vi "parse.vi"(8 "error in (no error)":errorcluster, 10 "ModbusBuffer in":refnum<class "ModbusBuffer.lvclass">, 11 "ILCCommunications in":refnum<class "ILCCommunications.lvclass">) -> (0 "error out":errorcluster, 2 "ModbusBuffer out":refnum<class "ModbusBuffer.lvclass">, 3 "ILCCommunications out":refnum<class "ILCCommunications.lvclass">)   [LabVIEW 2016, in "ILCCommunications.lvclass"]
uses:
  ILCCommunications.lvclass
  Common_RT_Modbus/ModbusBuffer/ModbusBuffer.lvclass
  Common_RT_Modbus/ModbusBuffer/ModbusBuffer.lvclass/ModbusBuffer.ctl
  ILCCommunications.lvclass/ILCCommunications.ctl
  Common_RT_ILC/ILC/ILC.lvclass/ILC.ctl
  Common_RT_HPILC/HPILC/HPILC.lvclass/HPILC.ctl
  Common_RT_FAILC/FAILC/FAILC.lvclass/FAILC.ctl
  Common_RT_Modbus/ModbusBuffer/readInstructionByte.vi
  getILCMap.vi
  Common_RT_ILC/ILC/parseILC.vi
  Common_RT_HPILC/HPILC/parseStepMotorResponse.vi
  Common_RT_HPILC/HPILC/parseStepMotorError.vi
  Common_RT_HPILC/HPILC/parseForceAndStatusResponse.vi
  Common_RT_HPILC/HPILC/parseForceAndStatusError.vi
  Common_RT_FAILC/FAILC/parseBoosterValveGainResponse.vi
  Common_RT_FAILC/FAILC/parseBoosterValveGainError.vi
  Common_RT_FAILC/FAILC/parseReadBoosterValveGainResponse.vi
  Common_RT_FAILC/FAILC/parseReadBoosterValveGainError.vi
  Common_RT_FAILC/FAILC/parseSetForceResponse.vi
  Common_RT_FAILC/FAILC/parseSetForceError.vi
  Common_RT_FAILC/FAILC/parseForceAndStatusResponse.vi
  Common_RT_FAILC/FAILC/parseForceAndStatusError.vi
  Common_RT_ILC/ILC/parseReportServerIDFrame.vi
  Common_RT_ILC/ILC/parseReportServerIDError.vi
  Common_RT_ILC/ILC/parseReportServerStatusFrame.vi
  Common_RT_ILC/ILC/parseReportServerStatusError.vi
  Common_RT_ILC/ILC/parseModeFrame.vi
  Common_RT_ILC/ILC/parseModeError.vi
  Common_RT_ILC/ILC/parseTemporaryAddressFrame.vi
  Common_RT_ILC/ILC/parseTemporaryAddressError.vi
  Common_RT_ILC/ILC/parseADCScanRateFrame.vi
  Common_RT_ILC/ILC/parseADCScanRateError.vi
  Common_RT_ILC/ILC/parseADCOffsetSensitivityFrame.vi
  Common_RT_ILC/ILC/parseADCOffsetSensitivityError.vi
  Common_RT_ILC/ILC/parseResetFrame.vi
  Common_RT_ILC/ILC/parseResetError.vi
  Common_RT_ILC/ILC/parseReportCalibrationDataFrame.vi
  Common_RT_ILC/ILC/parseReportCalibrationDataError.vi
  Common_RT_Modbus/ModbusBuffer/calculateCRC.vi
  Common_RT_Modbus/ModbusBuffer/readCRC.vi
  Common_RT_Modbus/ModbusBuffer/readTimestamp.vi
  Common_RT_Modbus/ModbusBuffer/readEndOfFrame.vi
  Common_RT_Modbus/ModbusBuffer/readI32.vi
  Common_RT_Modbus/ModbusBuffer/readSGL.vi
  Common_RT_Modbus/ModbusBuffer/readU48.vi
  Common_RT_Modbus/ModbusBuffer/readString.vi
  Common_RT_Modbus/ModbusBuffer/readU16.vi
  Common_RT_Modbus/ModbusBuffer/readTimestampByte.vi
  Common_RT_HPILC/HPILC/HPILC.lvclass
  D:/Code/ts_M1M3Support/Common_RT_ILC/ILC/ILC.lvclass
  Common_RT_FAILC/FAILC/FAILC.lvclass
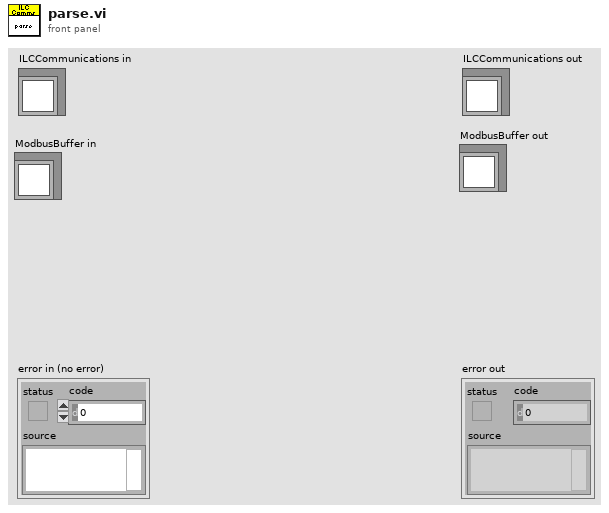
[diagram p1: front panel]
types:
  T1 = typedef "M1M3SupportGeneral.lvlib/ILCMap.ctl" = cluster{"Index":i32, "Type":T2}
  T2 = typedef "M1M3SupportGeneral.lvlib/ILCTypes.ctl" = enum16{"Hardpoint", "Force"}
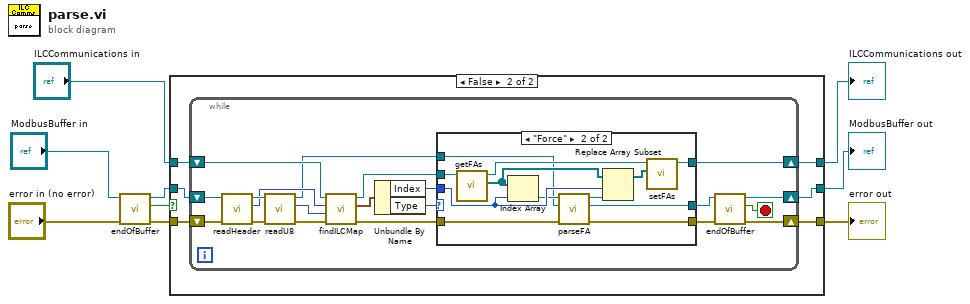
[diagram p0: block diagram]
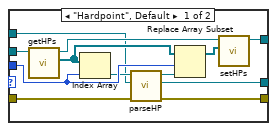
[diagram p3: hidden frame]
diagram:
  n1 = call "endOfBuffer.vi"("error in (no error)"="error in (no error)", "ModbusBuffer in"="ModbusBuffer in") -> ("error out"=w5:errorcluster, "EndOfBuffer"=w8:bool, "ModbusBuffer out"=w7:refnum<class "ModbusBuffer.lvclass">)  [unwired: 7 in]
  n2 = case shown="False" w8 {
    tunnel: w7 -> [w12 w17]
    tunnel: w5 -> [w11 w18]
    tunnel: [w12 w16] -> w4
    tunnel: [w11 w15] -> w3
    tunnel: "ILCCommunications in" -> [w10 w14]
    tunnel: [w10 w13] -> w1
    frame True {
    }
    frame False {
      n3 = while {
        shift-right: [w37] -> w15
        shift-left: w18 -> [w34]
        shift-right: [w36] -> w16
        shift-left: w17 -> [w35]
        shift-right: [w19] -> w13
        shift-left: w14 -> [w31]
        stop <- w38 stop-if-true
        n4 = call "readHeader.vi"("error in (no error)"=w34, "ModbusBuffer in"=w35) -> ("error out"=w32:errorcluster, "Subnet"=w30:u8, "ModbusBuffer out"=w33:refnum<class "ModbusBuffer.lvclass">)  [unwired: 6 in, 1 out]
        n5 = call "readU8.vi"("error in (no error)"=w32, "ModbusBuffer in"=w33) -> ("error out"=w28:errorcluster, "Output"=w29:u8, "ModbusBuffer out"=w23:refnum<class "ModbusBuffer.lvclass">)  [unwired: 7 in]
        n6 = call "findILCMap.vi"("error in (no error)"=w28, "Address"=w29, "Subnet"=w30, "ILCCommunications in"=w31) -> ("error out"=w21:errorcluster, "Map"=w27:T1, "ILCCommunications out"=w24:refnum<class "ILCCommunications.lvclass">)  [unwired: 5 in]
        n7 = Unbundle By Name(w27) -> ("Index"=w25:i32, "Type"=w26:T2)
        n8 = case shown="\"Force\"" w26 {
          tunnel: w25 -> [w46 w62]
          tunnel: w24 -> [w50 w54]
          tunnel: w23 -> [w43 w53]
          tunnel: [w42 w52] -> w22
          tunnel: w21 -> [w41 w60]
          tunnel: [w40 w59] -> w20
          tunnel: [w39 w51] -> w19
          frame "Hardpoint", Default {
            n9 = call "getHPs.vi"("ILCCommunications in"=w50) -> ("HPs"=w48:refnum<class "HPILC.lvclass">[], "ILCCommunications out"=w49:refnum<class "ILCCommunications.lvclass">)  [unwired: 9 in]
            n10 = Index Array(array=w48, index=w46) -> (element=w45:refnum<class "HPILC.lvclass">)
            n11 = call "parseHP.vi"("error in (no error)"=w41, "ModbusBuffer in"=w43, "HPILC in"=w45) -> ("error out"=w40:errorcluster, "ModbusBuffer out"=w42:refnum<class "ModbusBuffer.lvclass">, "HPILC out"=w44:refnum<class "HPILC.lvclass">)  [unwired: 5 in, 1 out]
            n12 = Replace Array Subset(array=w48, new element=w44, index=w46) -> (w47:refnum<class "HPILC.lvclass">[])
            n13 = call "setHPs.vi"("HPs"=w47, "ILCCommunications in"=w49) -> ("ILCCommunications out"=w39:refnum<class "ILCCommunications.lvclass">)  [unwired: 9 in]
          }
          frame "Force" {
            n14 = call "getFAs.vi"("ILCCommunications in"=w54) -> ("FAs"=w57:refnum<class "FAILC.lvclass">[], "ILCCommunications out"=w55:refnum<class "ILCCommunications.lvclass">)  [unwired: 9 in]
            n15 = Index Array(array=w57, index=w62) -> (element=w61:refnum<class "FAILC.lvclass">)
            n16 = call "parseFA.vi"("error in (no error)"=w60, "ModbusBuffer in"=w53, "FAILC in"=w61) -> ("error out"=w59:errorcluster, "ModbusBuffer out"=w52:refnum<class "ModbusBuffer.lvclass">, "FAILC out"=w58:refnum<class "FAILC.lvclass">)  [unwired: 5 in, 1 out]
            n17 = Replace Array Subset(array=w57, new element=w58, index=w62) -> (w56:refnum<class "FAILC.lvclass">[])
            n18 = call "setFAs.vi"("FAs"=w56, "ILCCommunications in"=w55) -> ("ILCCommunications out"=w51:refnum<class "ILCCommunications.lvclass">)  [unwired: 9 in]
          }
        }
        n19 = call "endOfBuffer.vi"("error in (no error)"=w20, "ModbusBuffer in"=w22) -> ("error out"=w37:errorcluster, "EndOfBuffer"=w38:bool, "ModbusBuffer out"=w36:refnum<class "ModbusBuffer.lvclass">)  [unwired: 7 in]
      }
    }
  }
  "error out" <- w3
  "ILCCommunications out" <- w1
  "ModbusBuffer out" <- w4
